vi "TagNameAndTypes.vi"() -> ()   [LabVIEW 2017]
uses:
  _lib/PQ/Taiko/PDLM_Tag.ctl
panel:
  in  "Tag":T1 items=["Locked"=16, "SoftLock"=17, "KeyLock"=18, "Class_IV_Lock"=20, "Interlock"=24, "LaserMode"=32, "TriggerMode"=48, "TriggerLevelRaw"=64, "TriggerLevelRawLoLimit"=65, "TriggerLevelRawHiLimit"=66, "TriggerLevel"=72, "TriggerLevelLoLimit"=73, "TriggerLevelHiLimit"=74, "FastGate"=80, "FastGateImp"=96, "SlowGate"=112, "TargetTempRaw"=144, "TargetTempRawLoLimit"=145, "TargetTempRawHiLimit"=146, "CurrentTempRaw"=148, "CaseTempRaw"=149, "TargetTemp"=152, "TargetTempLoLimit"=153, "TargetTempHiLimit"=154, "CurrentTemp"=156, "CaseTemp"=157, "TempScale"=159, "Frequency"=168, "FrequencyLoLimit"=169, "FrequencyHiLimit"=170, "PulsePowerRaw"=176, "PulsePowerRawLoLimit"=177, "PulsePowerRawHiLimit"=178, "PulsePowerPermille"=180, "PulseShape"=181, "PulsePower"=184, "PulsePowerLoLimit"=185, "PulsePowerHiLimit"=186, "PulsePowerNanowatt"=188, "PulsePowerVoltage"=190, "PulseEnergy"=191, "CwPowerRaw"=192, "CwPowerRawLoLimit"=193, "CwPowerRawHiLimit"=194, "CwPowerPermille"=196, "CwPower"=200, "CwPowerLoLimit"=201, "CwPowerHiLimit"=202, "CwPowerMicroWatt"=204, "BurstLen"=208, "BurstPeriod"=224, "LDH_Fan"=240, "UI_Exclusive"=256]
  out "NumTags":i32=53
  out "Tags":cluster{i32, "TypeCode":u32, "Name":string}[](array[cluster])=[{16, "TypeCode"=1, "Name"="Locked"}, {17, "TypeCode"=1, "Name"="SoftLock"}, {18, "TypeCode"=1, "Name"="KeyLock"}, {20, "TypeCode"=1, "Name"="Class_IV_Lock"}, {24, "TypeCode"=1, "Name"="Interlock"}, {32, "TypeCode"=65538, "Name"="LaserMode"}, {48, "TypeCode"=65538, "Name"="TriggerMode"}, {64, "TypeCode"=65539, "Name"="TriggerLevelRaw"}, {65, "TypeCode"=65539, "Name"="TriggerLevelRawLoLimit"}, {66, "TypeCode"=65539, "Name"="TriggerLevelRawHiLimit"}, {72, "TypeCode"=1114882, "Name"="TriggerLevel"}, {73, "TypeCode"=1114882, "Name"="TriggerLevelLoLimit"}, {74, "TypeCode"=1114882, "Name"="TriggerLevelHiLimit"}, {80, "TypeCode"=1, "Name"="FastGate"}, {96, "TypeCode"=65538, "Name"="FastGateImp"}, {112, "TypeCode"=1, "Name"="SlowGate"}, {144, "TypeCode"=65793, "Name"="TargetTempRaw"}, {145, "TypeCode"=65793, "Name"="TargetTempRawLoLimit"}, {146, "TypeCode"=65793, "Name"="TargetTempRawHiLimit"}, {148, "TypeCode"=65793, "Name"="CurrentTempRaw"}, {149, "TypeCode"=65793, "Name"="CaseTempRaw"}, {152, "TypeCode"=16777217, "Name"="TargetTemp"}, {153, "TypeCode"=16777217, "Name"="TargetTempLoLimit"}, {154, "TypeCode"=16777217, "Name"="TargetTempHiLimit"}, {156, "TypeCode"=16777217, "Name"="CurrentTemp"}, {157, "TypeCode"=16777217, "Name"="CaseTemp"}, {159, "TypeCode"=65538, "Name"="TempScale"}, {168, "TypeCode"=65537, "Name"="Frequency"}, {169, "TypeCode"=65537, "Name"="FrequencyLoLimit"}, {170, "TypeCode"=65537, "Name"="FrequencyHiLimit"}, {176, "TypeCode"=65539, "Name"="PulsePowerRaw"}, {177, "TypeCode"=65539, "Name"="PulsePowerRawLoLimit"}, {178, "TypeCode"=65539, "Name"="PulsePowerRawHiLimit"}, {180, "TypeCode"=66305, "Name"="PulsePowerPermille"}, {181, "TypeCode"=65538, "Name"="PulseShape"}, {184, "TypeCode"=16777217, "Name"="PulsePower"}, {185, "TypeCode"=67841, "Name"="PulsePowerLoLimit"}, {186, "TypeCode"=67841, "Name"="PulsePowerHiLimit"}, {188, "TypeCode"=67841, "Name"="PulsePowerNanowatt"}, {190, "TypeCode"=66306, "Name"="PulsePowerVoltage"}, {191, "TypeCode"=69377, "Name"="PulseEnergy"}, {192, "TypeCode"=65539, "Name"="CwPowerRaw"}, {193, "TypeCode"=65539, "Name"="CwPowerRawLoLimit"}, {194, "TypeCode"=65539, "Name"="CwPowerRawHiLimit"}, {196, "TypeCode"=66305, "Name"="CwPowerPermille"}, {200, "TypeCode"=16777217, "Name"="CwPower"}, {201, "TypeCode"=16777217, "Name"="CwPowerLoLimit"}, {202, "TypeCode"=16777217, "Name"="CwPowerHiLimit"}, {204, "TypeCode"=67073, "Name"="CwPowerMicroWatt"}, {208, "TypeCode"=65537, "Name"="BurstLen"}, {224, "TypeCode"=65537, "Name"="BurstPeriod"}, {240, "TypeCode"=1, "Name"="LDH_Fan"}, {256, "TypeCode"=1, "Name"="UI_Exclusive"}] {"?" format="%x"; "TypeCode" format="%x"}
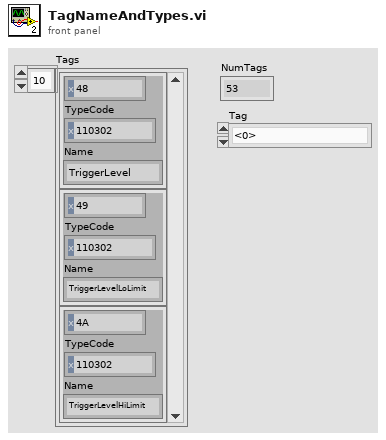
[diagram p1: front panel]
types:
  T1 = typedef "PDLM_Tag.ctl" = u32
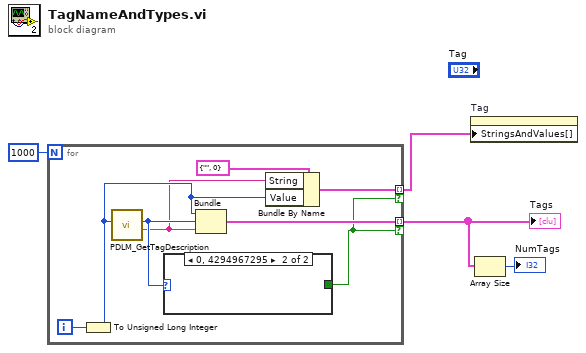
[diagram p0: block diagram]
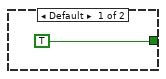
[diagram p2: hidden frame]
diagram:
  n1 = for {
    N: 1000 -> [_]
    tunnel: [w12] -> w3 mode=indexing if=w6
    tunnel: [w7] -> w1 mode=indexing if=w6
    i -> [w9]
    n2 = To Unsigned Long Integer(number=w9) -> (unsigned 32bit integer=w8:u32)
    n3 = call "PDLM_GetTagDescription.vi"("Tag"=w8) -> ("Name"=w5:string, "TypeCode"=w11:u32)  [unwired: 7 in, 2 out]
    n4 = case shown="0, 4294967295" w11 {
      tunnel: [TRUE _] -> w6
      frame Default {
      }
      frame 0, -1 {
      }
    }
    n5 = Bundle(w8, "TypeCode"=w11, "Name"=w5) -> (w12:cluster{u32, "TypeCode":u32, "Name":string})  [unwired: 1 in]
    n6 = Bundle By Name(cluster=cluster{"String":string, "Value":u32} {"String"="", "Value"=0} ("element"), "String"=w5, "Value"=w8) -> (w7:cluster{"String":string, "Value":u32})
  }
  "Tags" <- w3
  n7 = property on="Tag" class="Ring (strict)"("StringsAndValues[]"=w1) -> ()  [unwired: 2 in, 2 out]
  n8 = Array Size(array=w3) -> (size(s)=→"NumTags":i32)
